vi "CAN Receive.vi"(8 "error in (no error)":errorcluster, 9 "timeoutMs":u32=100, 10 "Message ID":u32 format="%.0x") -> (0 "error out":errorcluster, 1 "data":u8[](array[numeric]), 2 "Message ID Out":u32)   [LabVIEW 2009, in "CAN.lvlib"]
uses:
  CAN.lvlib
  Serial.lvlib
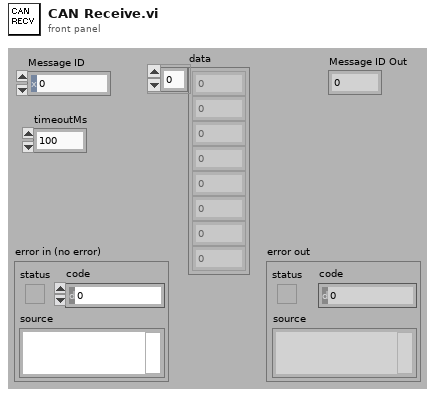
[diagram p1: front panel]
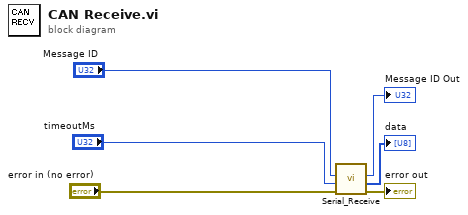
[diagram p0: block diagram]
diagram:
  n1 = call "Serial_Receive.vi"("error in (no error)"="error in (no error)", "timeoutMs"="timeoutMs", "Message ID"="Message ID") -> ("error out"=→"error out":errorcluster, "data"=→"data":u8[], "Message ID Out"=→"Message ID Out":u32)  [unwired: 3 in, 3 out]
